vi "S2C_PCIe7841_Proc_ConvertName.vi"(4 "Data In":string) -> (1 "Data Out":string)   [LabVIEW 2015]
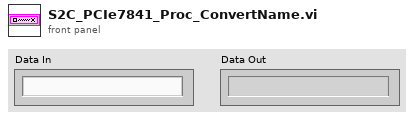
[diagram p1: front panel]
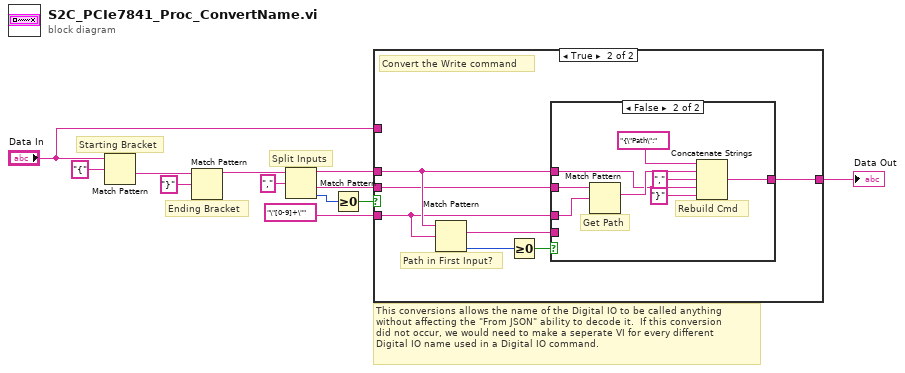
[diagram p0: block diagram]
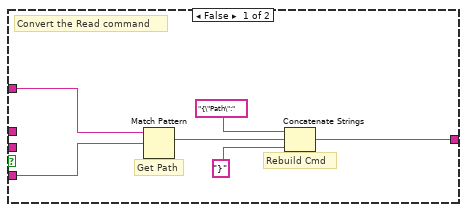
[diagram p2: hidden frame]
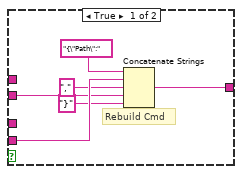
[diagram p3: hidden frame]
diagram:
  # "This conversions allows the name of the Digital IO to be called anything\nwithout affecting the \"From JSON\" ability to decode it.  If this conversion\ndid not occur, we would need to make a seperate VI for every different\nDigital IO name used in a Digital IO command."
  # "Split Inputs"
  # "Ending Bracket"
  # "Starting Bracket"
  n1 = Match Pattern(string="Data In", regular expression="{") -> (after substring=w10:string)  [unwired: 1 in, 3 out]
  n2 = Match Pattern(string=w10, regular expression="}") -> (before substring=w9:string)  [unwired: 1 in, 3 out]
  n3 = Match Pattern(string=w9, regular expression=",") -> (before substring=w7:string, after substring=w6:string, offset past match=w3:i32)  [unwired: 1 in, 1 out]
  n4 = Greater Or Equal To 0?(x=w3) -> (x >= 0?=w2:bool)
  n5 = case shown="True" w2 {
    tunnel: w7 -> [_ w23]
    tunnel: w6 -> [_ w22]
    tunnel: "\"[0-9]+\"" ("regular expression") -> [w17 w20]
    tunnel: [w13 w19] -> w4
    tunnel: "Data In" -> [w18 _]
    frame False {
      # "Convert the Read command"
      # "Rebuild Cmd"
      # "Get Path"
      n6 = Match Pattern(string=w18, regular expression=w17) -> (match substring=w15:string)  [unwired: 1 in, 3 out]
      n7 = Concatenate Strings("{\"Path\":", w15, "}") -> (w13:string)
    }
    frame True {
      # "Convert the Write command"
      # "Path in First Input?"
      n8 = Match Pattern(string=w23, regular expression=w20) -> (match substring=w21:string, offset past match=w25:i32)  [unwired: 1 in, 2 out]
      n9 = Greater Or Equal To 0?(x=w25) -> (x >= 0?=w24:bool)
      n10 = case shown="False" w24 {
        tunnel: w23 -> [_ w32]
        tunnel: w22 -> [w28 w34]
        tunnel: w21 -> [w30 _]
        tunnel: [w26 w36] -> w19
        tunnel: w20 -> [_ w35]
        frame True {
          # "Rebuild Cmd"
          n11 = Concatenate Strings("{\"Path\":" ("string"), w30, "," ("string"), w28, "}" ("string")) -> (w26:string)
        }
        frame False {
          # "Rebuild Cmd"
          # "Get Path"
          n12 = Match Pattern(string=w34, regular expression=w35) -> (match substring=w33:string)  [unwired: 1 in, 3 out]
          n13 = Concatenate Strings("{\"Path\":" ("string"), w33, "," ("string"), w32, "}" ("string")) -> (w36:string)
        }
      }
    }
  }
  "Data Out" <- w4
